vi "Get MC Test Data.vi"(4 "Actual refresh rate (ms)":u32, 5 "Initialise":bool, 6 "Initial Time Stamp":timestamp, 7 "Stop":bool, 8 "error in (no error)":errorcluster, 9 "MC Data montoring queue IN":refnum<queue>, 10 "MC Data queue IN":refnum<queue>, 11 "FPGA Ref in":T1) -> (0 "error out":errorcluster, 1 "MC state":enum16{"Waiting", "First frame", "Wrote Ref"}(ring))   [LabVIEW 2020]
uses:
  RIG-SPECIFIC FILES/FPGA Refs/FPGA Ref.ctl
  <vilib>/Utility/error.llb/Error Cluster From Error Code.vi
  <vilib>/rvi/errors/niLvFpgaAdjustHostInterfaceError.vi
  <vilib>/rvi/interface/nirviReadWriteControl/nirviReadWriteControl.xnode
  NiFpgaLv.dll
  <vilib>/rvi/interface/Simulation/niFpgaSimulationCallBeginRW.vi
panel:
  out "num_xyref_pixels":u16
  out "numxyzpixels":u16
  out "y_offset 3":fxp<+/-,16,8>
  out "X_Y_Z":bool[](array[boolean])
  out "MC state 2":enum16{"Waiting", "First frame", "Wrote Ref"}(ring)
  out "y_offset 2":fxp<+/-,16,8>
  out "y_offset":fxp<+/-,16,8>
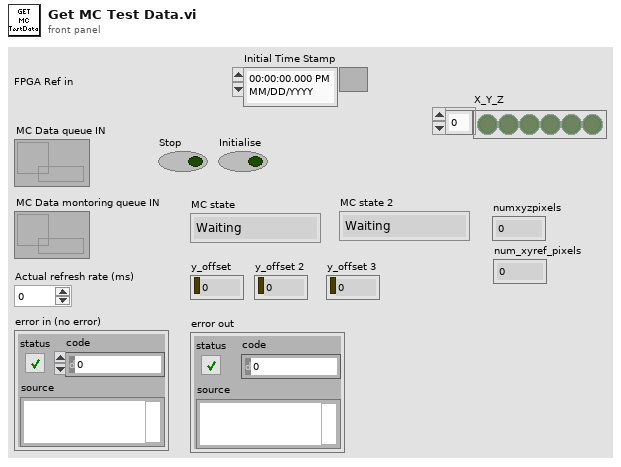
[diagram p1: front panel]
types:
  T1 = typedef "FPGA Ref.ctl" = refnum<k20>
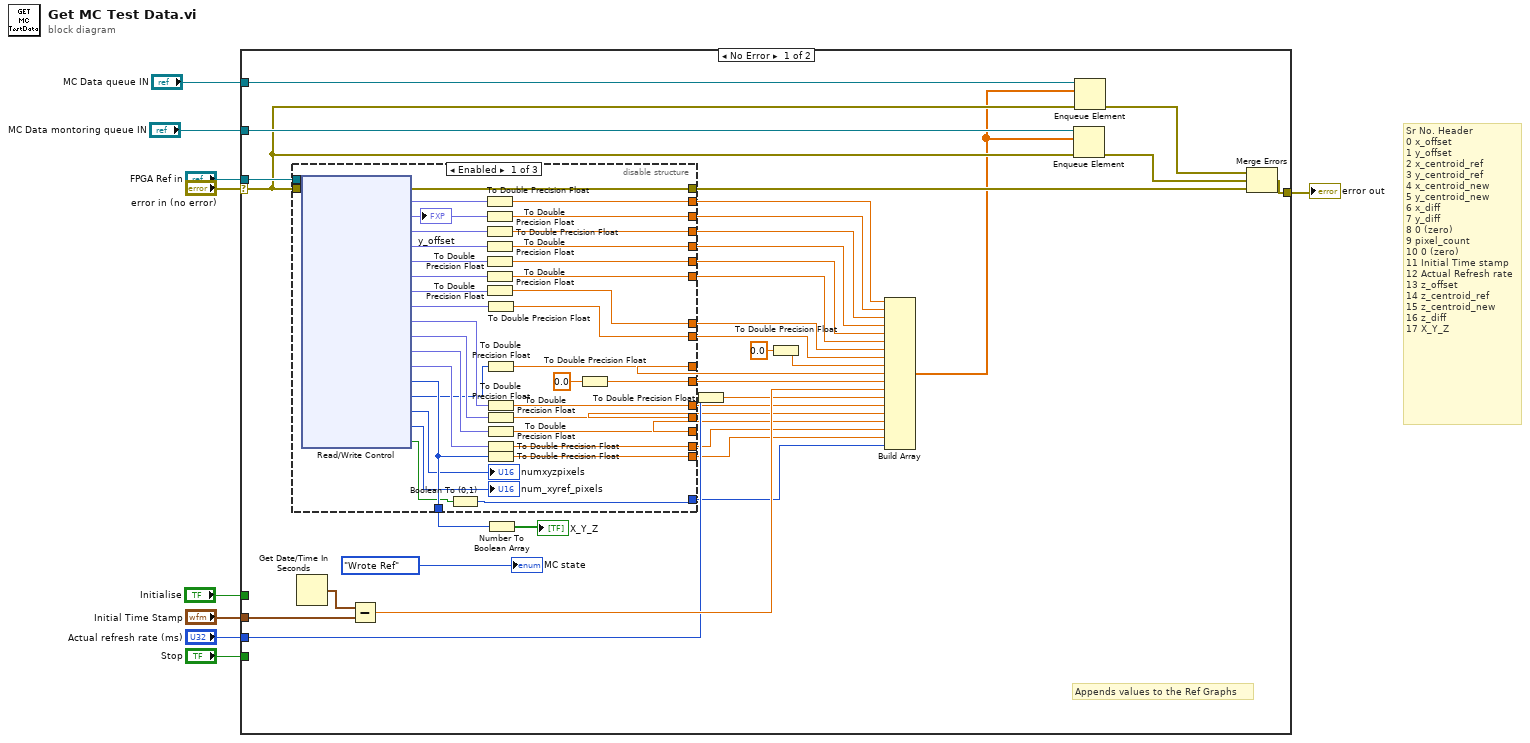
[diagram p0: block diagram]
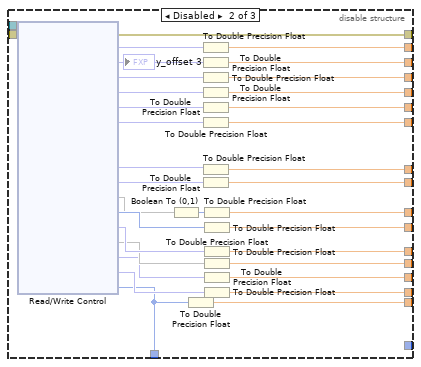
[diagram p2: hidden frame]
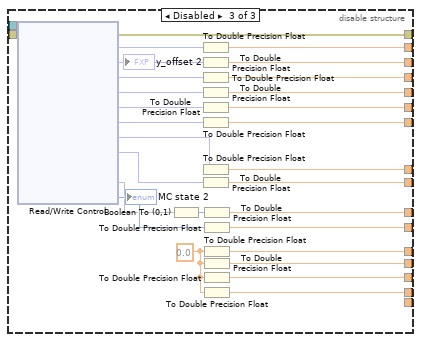
[diagram p3: hidden frame]
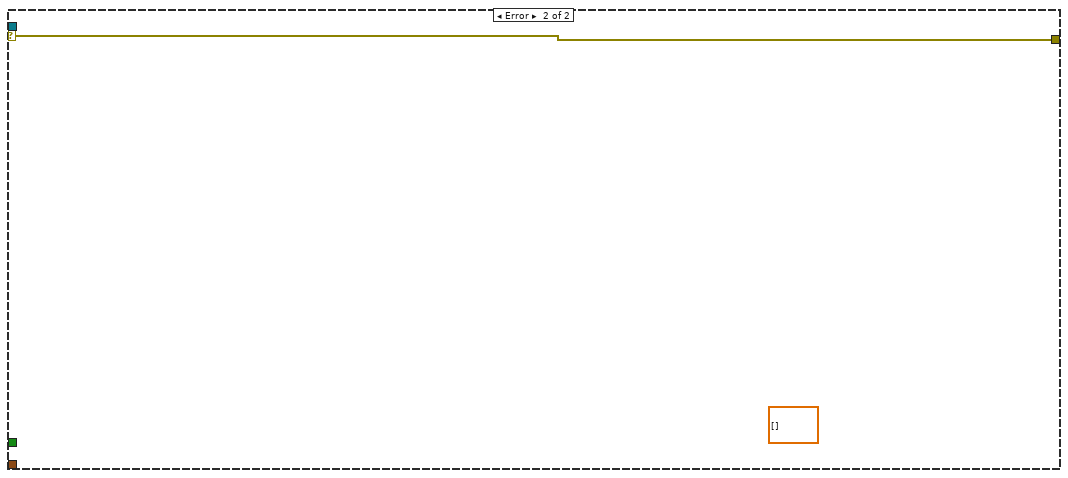
[diagram p4: hidden frame]
diagram:
  # "Sr No.\tHeader\n0\tx_offset\n1\ty_offset\n2\tx_centroid_ref\n3\ty_centroid_ref\n4\tx_centroid_new\n5\ty_centroid_new\n6\tx_diff\n7\ty_diff\n8\t0 (zero)\n9\tpixel_count\n10\t0 (zero)\n11\tInitial Time stamp\n12\tActual Refresh rate\n13\tz_offset\n14\tz_centroid_ref\n15\tz_centroid_new\n16\tz_diff\n17\tX_Y_Z"
  n1 = case shown="No Error" "error in (no error)" {
    selector: "error in (no error)" -> [w13 w146]
    tunnel: "FPGA Ref in" -> [w44 _]
    tunnel: "Initial Time Stamp" -> [w32 _]
    tunnel: [w30 w146] -> w6
    tunnel: "Actual refresh rate (ms)" -> [w27 _]
    tunnel: "Stop" -> [_ _]
    tunnel: "Initialise" -> [_ _]
    tunnel: "MC Data queue IN" -> [w15 _]
    tunnel: "MC Data montoring queue IN" -> [w14 _]
    frame No Error {
      # "Appends values to the Ref Graphs"
      n2 = disable-structure shown="Enabled" {
        disable-tunnel: w44 -> [w81 w115 w145]
        disable-tunnel: [w80 w113 w143] -> w43
        disable-tunnel: [w79 w112 w142] -> w42
        disable-tunnel: [w78 w109 w139] -> w40
        disable-tunnel: [w77 w108 w138] -> w39
        disable-tunnel: [w76 w107 w137] -> w38
        disable-tunnel: [w75 w106 w136] -> w37
        disable-tunnel: [w74 w105 w135] -> w36
        disable-tunnel: [w73 w104 w134] -> w35
        disable-tunnel: [w72 w103 w133] -> w34
        disable-tunnel: [w71 w102 w132] -> w33
        disable-tunnel: w13 -> [w62 w93 w122]
        disable-tunnel: [w61 w92 w121] -> w29
        disable-tunnel: [w48 w90 w120] -> w26
        disable-tunnel: [w56 w86 w119] -> w22
        disable-tunnel: [w55 w85 w118] -> w25
        disable-tunnel: [w54 w84 w117] -> w24
        disable-tunnel: [w53 w83 _] -> w21
        disable-tunnel: [w52 w82 _] -> w20
        disable-tunnel: [w45 _ _] -> w16
        frame Enabled {
          n3 = xnode "Read/Write Control"("FPGA VI Reference In"=w81, "error in"=w62) -> ("error out"=w61:errorcluster, "x_offset"=w69:fxp<+/-,16,8>, "y_offset"=w67:fxp<+/-,16,8>, "x_centroid_ref"=w63:fxp<+,32,16>, "y_centroid_ref"=w64:fxp<+,32,16>, "x_centroid_new"=w65:fxp<+,32,16>, "y_centroid_new"=w66:fxp<+,32,16>, "x_diff"=w68:fxp<+/-,16,8>, "y_diff"=w70:fxp<+/-,16,8>, "z offset"=w60:fxp<+/-,16,8>, "z_centroid_ref"=w59:fxp<+,32,16>, "z_centroid_new"=w57:fxp<+,32,16>, "z_diff"=w58:fxp<+/-,16,8>, "X_Y_Z"=w52:u64, "pixel_count"=w51:u16, "numxyzpixels"=→"numxyzpixels":u16, "num_xyref_pixels"=→"num_xyref_pixels":u16, "background_mc"=w46:bool)  [unwired: 1 out]
          "y_offset" <- w67
          n4 = Boolean To (0,1)(Boolean=w46) -> (0, 1=w45:i16)
          n5 = To Double Precision Float(number=w69) -> (double precision float=w78:dbl)
          n6 = To Double Precision Float(number=w67) -> (double precision float=w71:dbl)
          n7 = To Double Precision Float(number=w63) -> (double precision float=w72:dbl)
          n8 = To Double Precision Float(number=w64) -> (double precision float=w73:dbl)
          n9 = To Double Precision Float(number=w65) -> (double precision float=w74:dbl)
          n10 = To Double Precision Float(number=w66) -> (double precision float=w75:dbl)
          n11 = To Double Precision Float(number=w68) -> (double precision float=w76:dbl)
          n12 = To Double Precision Float(number=w70) -> (double precision float=w77:dbl)
          n13 = To Double Precision Float(number=w51) -> (double precision float=w79:dbl)
          n14 = To Double Precision Float(number=w60) -> (double precision float=w48:dbl)
          n15 = To Double Precision Float(number=w59) -> (double precision float=w56:dbl)
          n16 = To Double Precision Float(number=w57) -> (double precision float=w55:dbl)
          n17 = To Double Precision Float(number=w58) -> (double precision float=w54:dbl)
          n18 = To Double Precision Float(number=w52) -> (double precision float=w53:dbl)
          n19 = To Double Precision Float(number=0.0) -> (double precision float=w80:dbl)
        }
        frame Disabled {
          n20 = xnode "Read/Write Control"("FPGA VI Reference In"=w115, "error in"=w93) -> ("error out"=w92:errorcluster, "x_offset"=w100:fxp<+/-,16,8>, "y_offset"=w98:fxp<+/-,16,8>, "x_centroid_ref"=w94:fxp<+,32,16>, "y_centroid_ref"=w95:fxp<+,32,16>, "x_centroid_new"=w96:fxp<+,32,16>, "y_centroid_new"=w97:fxp<+,32,16>, "x_diff"=w99:fxp<+/-,16,8>, "y_diff"=w101:fxp<+/-,16,8>, "_SS"=w110, "Data Out"=w114:u64, "z offset"=w91:fxp<+/-,16,8>, "z_centroid_ref"=w89, "z_centroid_new"=w87:fxp<+,32,16>, "z_diff"=w88:fxp<+/-,16,8>, "X_Y_Z"=w82:u64)  [unwired: 3 out]
          "y_offset 3" <- w98
          n21 = Boolean To (0,1)(Boolean=w110) -> (0, 1=w111:i16)
          n22 = To Double Precision Float(number=w82) -> (double precision float=w83:dbl)
          n23 = To Double Precision Float(number=w100) -> (double precision float=w109:dbl)
          n24 = To Double Precision Float(number=w98) -> (double precision float=w102:dbl)
          n25 = To Double Precision Float(number=w94) -> (double precision float=w103:dbl)
          n26 = To Double Precision Float(number=w95) -> (double precision float=w104:dbl)
          n27 = To Double Precision Float(number=w96) -> (double precision float=w105:dbl)
          n28 = To Double Precision Float(number=w97) -> (double precision float=w106:dbl)
          n29 = To Double Precision Float(number=w99) -> (double precision float=w107:dbl)
          n30 = To Double Precision Float(number=w101) -> (double precision float=w108:dbl)
          n31 = To Double Precision Float(number=w111) -> (double precision float=w112:dbl)
          n32 = To Double Precision Float(number=w114) -> (double precision float=w113:dbl)
          n33 = To Double Precision Float(number=w91) -> (double precision float=w90:dbl)
          n34 = To Double Precision Float(number=w89) -> (double precision float=w86:dbl)
          n35 = To Double Precision Float(number=w87) -> (double precision float=w85:dbl)
          n36 = To Double Precision Float(number=w88) -> (double precision float=w84:dbl)
        }
        frame Disabled {
          w116 = 0.0
          n37 = xnode "Read/Write Control"("FPGA VI Reference In"=w145, "error in"=w122) -> ("error out"=w121:errorcluster, "x_offset"=w130:fxp<+/-,16,8>, "y_offset"=w128:fxp<+/-,16,8>, "x_centroid_ref"=w123:fxp<+,32,16>, "y_centroid_ref"=w124:fxp<+,32,16>, "x_centroid_new"=w125:fxp<+,32,16>, "y_centroid_new"=w126:fxp<+,32,16>, "x_diff"=w129:fxp<+/-,16,8>, "y_diff"=w131:fxp<+/-,16,8>, "MC State"=→"MC state 2", "_SS"=w140, "Data Out"=w144:u64)  [unwired: 1 out]
          "y_offset 2" <- w128
          n38 = Boolean To (0,1)(Boolean=w140) -> (0, 1=w141:i16)
          n39 = To Double Precision Float(number=w130) -> (double precision float=w139:dbl)
          n40 = To Double Precision Float(number=w128) -> (double precision float=w132:dbl)
          n41 = To Double Precision Float(number=w123) -> (double precision float=w133:dbl)
          n42 = To Double Precision Float(number=w124) -> (double precision float=w134:dbl)
          n43 = To Double Precision Float(number=w125) -> (double precision float=w135:dbl)
          n44 = To Double Precision Float(number=w126) -> (double precision float=w136:dbl)
          n45 = To Double Precision Float(number=w129) -> (double precision float=w137:dbl)
          n46 = To Double Precision Float(number=w131) -> (double precision float=w138:dbl)
          n47 = To Double Precision Float(number=w141) -> (double precision float=w142:dbl)
          n48 = To Double Precision Float(number=w144) -> (double precision float=w143:dbl)
          n49 = To Double Precision Float(number=w116) -> (double precision float=w120:dbl)
          n50 = To Double Precision Float(number=w116) -> (double precision float=w119:dbl)
          n51 = To Double Precision Float(number=w116) -> (double precision float=w118:dbl)
          n52 = To Double Precision Float(number=w116) -> (double precision float=w117:dbl)
        }
      }
      n53 = Get Date/Time In Seconds() -> (seconds since 1Jan1904=w23:timestamp)
      n54 = Subtract(x=w23, y=w32) -> (x-y=w31:dbl)
      n55 = Number To Boolean Array(number=w20) -> (Boolean array=→"X_Y_Z":bool[])
      n56 = To Double Precision Float(number=w27) -> (double precision float=w28:dbl)
      n57 = To Double Precision Float(number=0.0) -> (double precision float=w41:dbl)
      n58 = Build Array(w40, w33, w34, w35, w36, w37, w38, w39, w41, w42, w43, w31, w28, w26, w22, w25, w24, w21, w16) -> (w12:dbl[])
      n59 = Enqueue Element(queue=w14, element=w12, error in (no error)=w13) -> (error out=w10:errorcluster)  [unwired: 1 in, 2 out]
      n60 = Enqueue Element(queue=w15, element=w12, error in (no error)=w13) -> (error out=w11:errorcluster)  [unwired: 1 in, 2 out]
      n61 = Merge Errors(w11, w10, w29) -> (w30:errorcluster)
      "MC state" <- enum16{"Waiting", "First frame", "Wrote Ref"}."Wrote Ref" ("MC state")
    }
    frame Error {
      (unwired) dbl[][] []
    }
  }
  "error out" <- w6
